vi "Open All Relays.vi"(9 "Device":string) -> (0 "error out":errorcluster)   [LabVIEW 2015]
uses:
  <vilib>/DAQmx/write.llb/DAQmx Write (Digital U32 1Chan 1Samp).vi
  <vilib>/DAQmx/create/channels.llb/DAQmx Create Channel (DO-Digital Output).vi
  <vilib>/DAQmx/miscellaneous.llb/DAQmx Fill In Error Info.vi
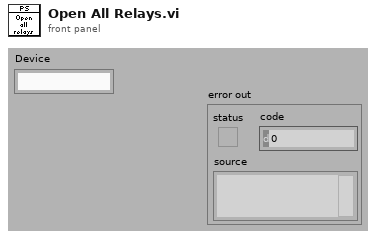
[diagram p1: front panel]
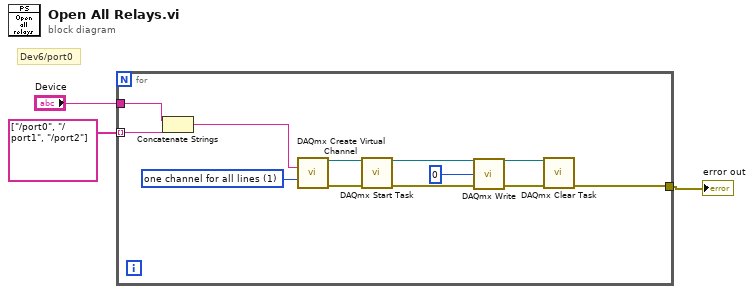
[diagram p0: block diagram]
diagram:
  # "Dev6/port0"
  n1 = for {
    tunnel: [w7] -> w3
    tunnel: string[] ["/port0", "/port1", "/port2"] ("Array") -> [w6] mode=indexing
    tunnel: "Device" -> [w5]
    w14 = 1 items=["one channel for each line", "one channel for all lines"] ("line grouping")
    n2 = Concatenate Strings(w5, w6) -> (w4:string)
    n3 = call-poly <vilib>:"DAQmx Create Virtual Channel.vi"("lines"=w4, "line grouping"=w14) -> ("task out"=w12:refnum<k21>, "error out"=w13:errorcluster)  [unwired: 12 in]
    n4 = call <vilib>:"DAQmx Start Task.vi"("task/channels in"=w12, "error in"=w13) -> ("task out"=w10:refnum<k21>, "error out"=w8:errorcluster)  [unwired: 12 in]
    n5 = call-poly <vilib>:"DAQmx Write.vi"("task/channels in"=w10, "data"=u32 0, "error in"=w8) -> ("task out"=w11:refnum<k21>, "error out"=w9:errorcluster)  [unwired: 10 in, 1 out]
    n6 = call <vilib>:"DAQmx Clear Task.vi"("task in"=w11, "error in"=w9) -> ("error out"=w7:errorcluster)  [unwired: 13 in]
  }
  "error out" <- w3
